vi "Core Action.vi"(8 "error in (no error)":errorcluster, 10 "SECS-II Class":refnum<class "SECS-II Class.lvclass">, 11 "29-Equipment Requests Time Value from Host in":refnum<class "29-Equipment Requests Time Value from Host.lvclass">) -> (0 "error out":errorcluster, 2 "SECS-II Class Out":refnum<class "SECS-II Class.lvclass">, 3 "29-Equipment Requests Time Value from Host out":refnum<class "29-Equipment Requests Time Value from Host.lvclass">)   [LabVIEW 2020, in "SECS Scenarios.lvlib" / "29-Equipment Requests Time Value from Host.lvclass"]
uses:
  29-Equipment Requests Time Value from Host.lvclass
  D:/Dropbox/SECS/SECS_GEM v1.1.0/Com/SECS Scenarios/Scenarios Class/Scenarios Class.lvclass
  SECS Communication/SECS-II Class/SECS-II Class.lvclass
  29-Equipment Requests Time Value from Host.lvclass/29-Equipment Requests Time Value from Host.ctl
  SECS Communication/S2 Message Class/S2 Message Class.lvclass
  D:/Dropbox/SECS/SECS_GEM v1.1.0/Com/SECS Communication/SECS-II Class/SECS-II Class.lvclass
  Scenarios Class/Scenarios Class.lvclass/Scenarios Class.ctl
  Scenarios Class/Reply State.ctl
  Scenarios Class/Write Reply State.vi
  Scenarios Class/Read HSMS Class.vi
  SECS Communication/HSMS Class/HSMS Class.lvclass
  Scenarios Class/Scenarios Class.lvclass
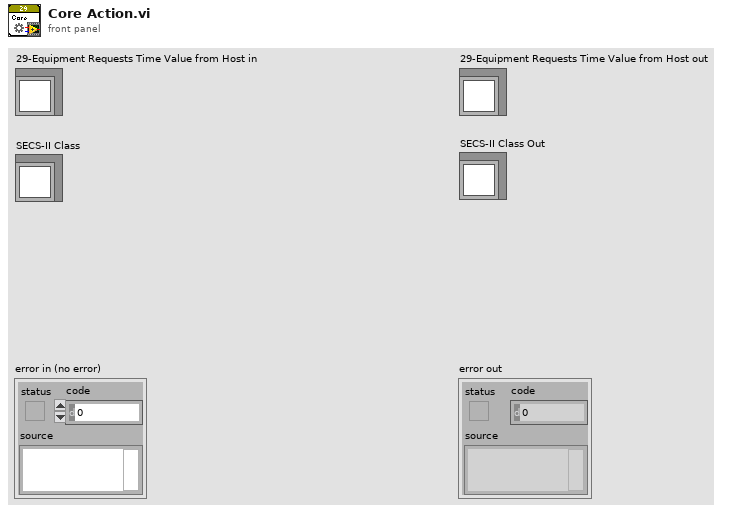
[diagram p1: front panel]
types:
  T1 = typedef "SECS Scenarios.lvlib/Scenarios Class.lvclass/Reply State.ctl" = enum16{"OK", "Illegal Data", "Unknown Stream", "Unknown Function", "Off-Line", "T3 Timeout", "Inner-Timeout"}
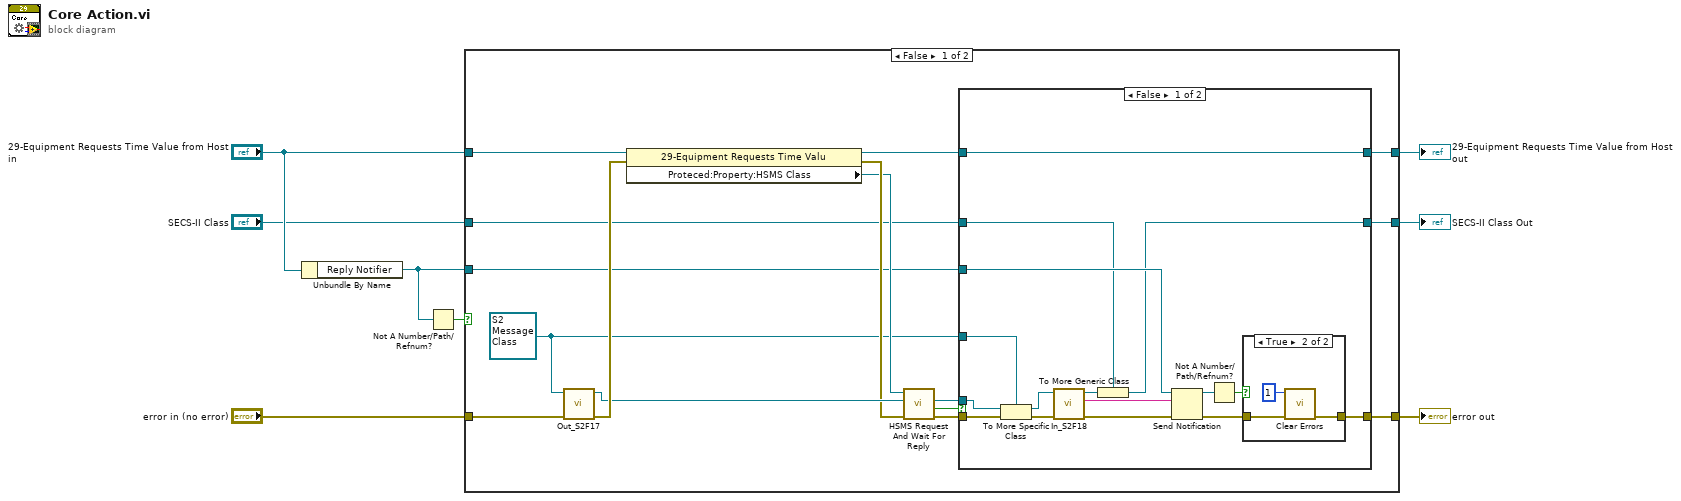
[diagram p0: block diagram]
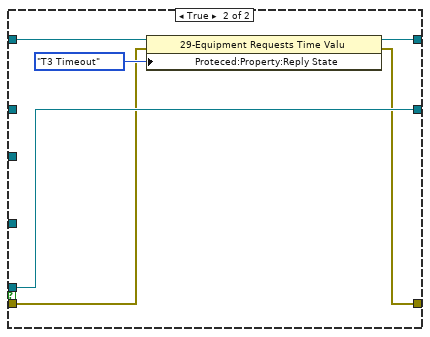
[diagram p3: hidden frame]
diagram:
  n1 = Unbundle By Name("29-Equipment Requests Time Value from Host in") -> ("Reply Notifier"=w7:refnum<notifier>)
  n2 = Not A Number/Path/Refnum?(number/path/refnum=w7) -> (NaN/Path/Refnum?=w8:bool)
  n3 = case shown="False" w8 {
    tunnel: w7 -> [w14 _]
    tunnel: "error in (no error)" -> [w24 w52]
    tunnel: "29-Equipment Requests Time Value from Host in" -> [w23 w53]
    tunnel: [w12 w53] -> w4
    tunnel: [w11 w52] -> w3
    tunnel: "SECS-II Class" -> [w10 w51]
    tunnel: [w9 w51] -> w1
    frame False {
      w15 = refnum<class "S2 Message Class.lvclass"> refnum ("S2 Message Class in")
      n4 = call "Out_S2F17.vi"("error in (no error)"=w24, "S2 Message Class in"=w15) -> ("error out"=w22:errorcluster, "S2 Message Class out"=w21:refnum<class "S2 Message Class.lvclass">)  [unwired: 8 in]
      n5 = property class="29-Equipment Requests Time Valu"(reference=w23, error in=w22) -> (reference out=w13:refnum<class "29-Equipment Requests Time Value from Host.lvclass">, error out=w20:errorcluster, "Proteced:Property:HSMS Class"=w19:refnum<class "HSMS Class.lvclass">)
      n6 = call "HSMS Request And Wait For Reply.vi"("error in (no error)"=w20, "SECS-II Class In"=w21, "HSMS Class in"=w19) -> ("error out"=w18:errorcluster, "Timeout?"=w17:bool, "SECS-II Class Out"=w16:refnum<class "SECS-II Class.lvclass">)  [unwired: 5 in, 1 out]
      n7 = case shown="False" w17 {
        tunnel: w18 -> [w40 w47]
        tunnel: w16 -> [w39 w50]
        tunnel: w15 -> [w38 _]
        tunnel: w14 -> [w33 _]
        tunnel: w13 -> [w32 w49]
        tunnel: [w32 w46] -> w12
        tunnel: [w28 w45] -> w11
        tunnel: w10 -> [w26 _]
        tunnel: [w25 w50] -> w9
        frame False {
          n8 = To More Specific Class(target class=w38, reference=w39, error in=w40) -> (specific class reference=w36:refnum<class "S2 Message Class.lvclass">, error out=w37:errorcluster)
          n9 = call "In_S2F18.vi"("error in (no error)"=w37, "S2 Message Class in"=w36) -> ("error out"=w35:errorcluster, "Time"=w34:string, "S2 Message Class out"=w27:refnum<class "S2 Message Class.lvclass">)  [unwired: 6 in, 1 out]
          n10 = To More Generic Class(target class=w26, reference=w27) -> (generic class reference=w25:refnum<class "SECS-II Class.lvclass">)
          n11 = Send Notification(notification=w34, notifier=w33, error in (no error)=w35) -> (notifier out=w31:refnum<notifier>, error out=w30:errorcluster)
          n12 = Not A Number/Path/Refnum?(number/path/refnum=w31) -> (NaN/Path/Refnum?=w29:bool)
          n13 = case shown="True" w29 {
            tunnel: w30 -> [w41 w43]
            tunnel: [w41 w42] -> w28
            frame False {
            }
            frame True {
              n14 = call <vilib>:"Clear Errors.vi"("error in (no error)"=w43, "specific error code to clear (0: all)"=1) -> ("error out"=w42:errorcluster)  [unwired: 4 in, 1 out]
            }
          }
        }
        frame True {
          n15 = property class="29-Equipment Requests Time Valu"(reference=w49, error in=w47, "Proteced:Property:Reply State"=Reply_State."T3 Timeout" ("Reply State")) -> (reference out=w46:refnum<class "29-Equipment Requests Time Value from Host.lvclass">, error out=w45:errorcluster)
        }
      }
    }
    frame True {
    }
  }
  "error out" <- w3
  "29-Equipment Requests Time Value from Host out" <- w4
  "SECS-II Class Out" <- w1
